vi "getWTInfo.vi"   [LabVIEW 2017]
uses:
  Controls/blocksWTInfo.ctl
  <vilib>/Analysis/baseanly.llb/Mean (DBL).vi
  Globals/measurementGlobal.vi
  <vilib>/Analysis/NI_AALBase.lvlib
types:
  T1 = typedef "blocksWTInfo.ctl" = cluster{"Velocity (ms^-1)":dbl, "Density (kgm^-3)":dbl, "Pressure (Pa)":dbl, "Temperature (K)":dbl}
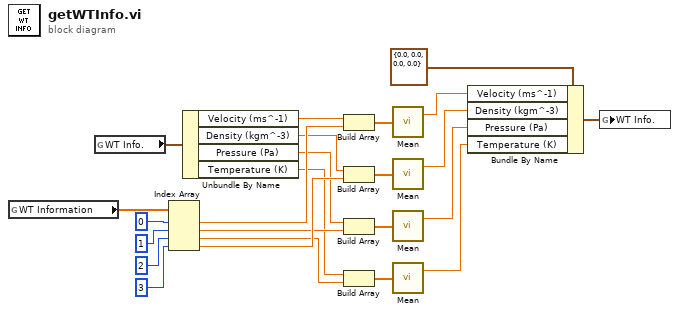
[diagram p0: block diagram]
diagram:
  n1 = global read "measurementGlobal.vi" "WT Information"() -> (w22:dbl[])
  n2 = global read "measurementGlobal.vi" "WT Info."() -> (w24:T1)
  n3 = Index Array(array=w22, index #1=0 ("index"), index #2=1 ("index"), index #3=2 ("index"), index #4=3 ("index")) -> (element #1=w15:dbl, element #2=w12:dbl, element #3=w9:dbl, element #4=w14:dbl)
  n4 = Unbundle By Name(w24) -> ("Velocity (ms^-1)"=w16:dbl, "Density (kgm^-3)"=w13:dbl, "Pressure (Pa)"=w11:dbl, "Temperature (K)"=w10:dbl)
  n5 = Build Array(w16, w15) -> (w8:dbl[])
  n6 = Build Array(w13, w14) -> (w7:dbl[])
  n7 = Build Array(w11, w12) -> (w6:dbl[])
  n8 = Build Array(w10, w9) -> (w5:dbl[])
  n9 = call-poly <vilib>:"Mean.vi"("X"=w8) -> ("mean"=w4:dbl)  [unwired: 1 out]
  n10 = call-poly <vilib>:"Mean.vi"("X"=w7) -> ("mean"=w3:dbl)  [unwired: 1 out]
  n11 = call-poly <vilib>:"Mean.vi"("X"=w6) -> ("mean"=w2:dbl)  [unwired: 1 out]
  n12 = call-poly <vilib>:"Mean.vi"("X"=w5) -> ("mean"=w1:dbl)  [unwired: 1 out]
  n13 = Bundle By Name(cluster=T1 {"Velocity (ms^-1)"=0.0, "Density (kgm^-3)"=0.0, "Pressure (Pa)"=0.0, "Temperature (K)"=0.0} ("WT Info."), "Velocity (ms^-1)"=w4, "Density (kgm^-3)"=w3, "Pressure (Pa)"=w2, "Temperature (K)"=w1) -> (w23:T1)
  n14 = global write "measurementGlobal.vi" "WT Info."(w23) -> ()
